vi "Event Nested Teardown.vi"(11 "Base Queue jettl in":refnum<class "Base Queue jettl.lvclass">) -> (3 "Base Queue jettl out":refnum<class "Base Queue jettl.lvclass">)   [LabVIEW 2021, in "jettl.lvlib" / "Base Queue jettl.lvlib" / "Base Queue jettl.lvclass"]
uses:
  Base Queue jettl.lvclass
  Msg Strategy/Teardown/Teardown Msg Strategy/Teardown Msg Strategy.lvclass
  C:/git/jettl/src/jettl/Msg Strategy/Msg Strategy/Msg Strategy.lvclass
  Base Queue jettl.lvclass/Base Queue jettl.ctl
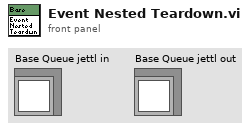
[diagram p1: front panel]
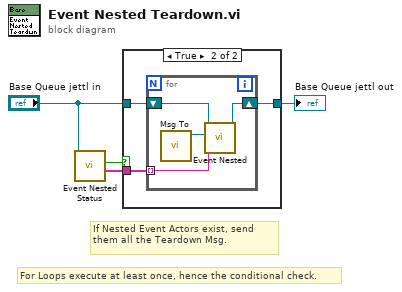
[diagram p0: block diagram]
diagram:
  # "If Nested Event Actors exist, send them all the Teardown Msg."
  # "For Loops execute at least once, hence the conditional check."
  n1 = call-dynamic "Event Nested Status.vi"("Base Queue jettl in"="Base Queue jettl in") -> ("Event Nested Aliases"=w3:string[], "Any Exist?"=w4:bool)  [unwired: 8 in, 1 out]
  n2 = case shown="True" w4 {
    tunnel: [w5 w8] -> w1
    tunnel: "Base Queue jettl in" -> [w5 w7]
    tunnel: w3 -> [_ w6]
    frame False {
    }
    frame True {
      n3 = for {
        tunnel: w6 -> [w9] mode=indexing
        shift-right: [w11] -> w8
        shift-left: w7 -> [w12]
        n4 = call "Msg To.vi"() -> ("Teardown Msg out"=w10:refnum<class "Teardown Msg Strategy.lvclass">)  [unwired: 11 in]
        n5 = call-dynamic "Event Nested.vi"("Alias"=w9, "Msg Strategy"=w10, "Base Queue jettl in"=w12) -> ("Base Queue jettl out"=w11:refnum<class "Base Queue jettl.lvclass">)  [unwired: 8 in]
      }
    }
  }
  "Base Queue jettl out" <- w1
